vi "Chart.vi"() -> (7 "Waveform Chart":dbl(graph))   [LabVIEW 2020]
doc: "This system is a subVI which is used to plot the data as per the value change in the slider in the main system"
panel:
  out "Error out":errorcluster
  in  "Error in":errorcluster
  # "Chart to Display data"
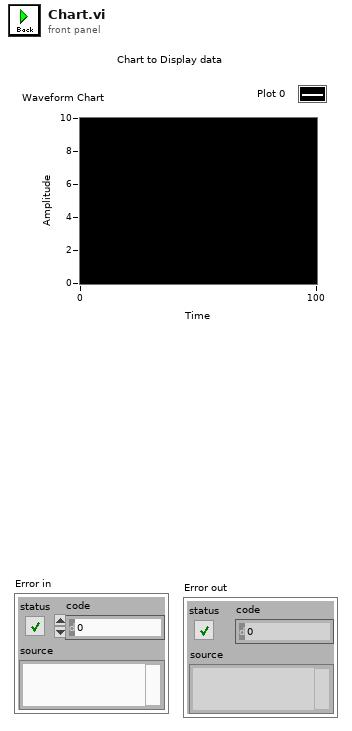
[diagram p1: front panel]
types:
  T1 = enum16{"Get Ref", "Destroy", "Create", "Generate"}
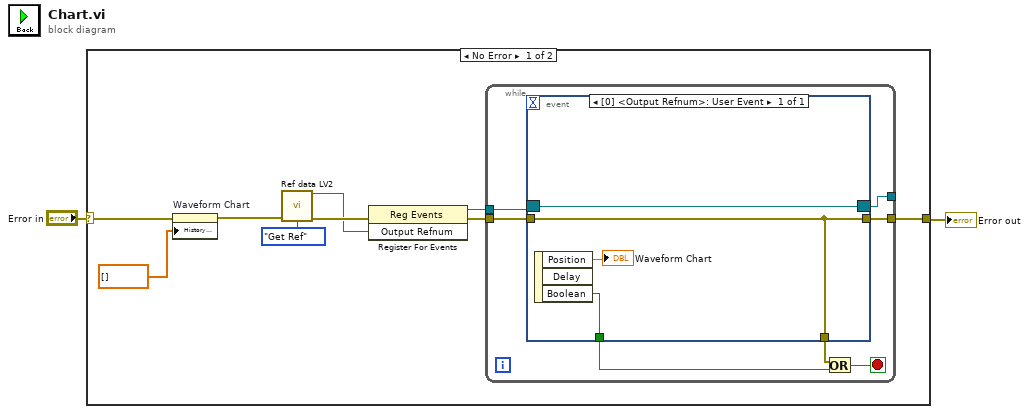
[diagram p0: block diagram]
diagram:
  n1 = case shown="No Error" "Error in" {
    selector: "Error in" -> [w5 w23]
    tunnel: [w6 w23] -> w1
    frame No Error {
      n2 = property on="Waveform Chart" class="WFChart (strict)"(error in=w5, "History Data"=dbl[] []) -> (error out=w4:errorcluster)  [unwired: 1 in, 1 out]
      n3 = call "Ref data LV2.vi"("error in"=w4, "Enum"=T1."Get Ref") -> ("Output Refnum"=w7:refnum<user-event>, "error out"=w11:errorcluster)  [unwired: 12 in]
      n4 = register-events(error in=w11, w7) -> (reference out=w8:refnum<event-registration>, error out=w9:errorcluster)  [unwired: 1 in]
      n5 = while {
        tunnel: w9 -> [w18]
        tunnel: [w17] -> w6
        tunnel: w8 -> [w16]
        tunnel: [w15] -> _
        stop <- w12 stop-if-true
        n6 = event shown="[0] <Output Refnum>: User Event" {
          selector: w16 -> [w21]
          dyn-events: [w21] -> w15
          timeout: _ -> [_]
          tunnel: w18 -> [w19]
          tunnel: [w19] -> w17
          tunnel: [w20] -> w14
          tunnel: [w19] -> w13
          event User Event {
            n7 = event-data() -> ("Position"=→"Waveform Chart":dbl, "Boolean"=w20:bool)  [unwired: 1 in, 1 out]
          }
        }
        n8 = Or(x=w13, y=w14) -> (x .or. y?=w12:bool)
      }
    }
    frame Error {
    }
  }
  "Error out" <- w1
